vi "Inversion Neighborhood.vi"(8 "w":i32, 9 "y":i32, 10 "Generate Random Indices?":bool, 11 "Schedule in":u16[](array[numeric])) -> (3 "Schedule out":u16[](array[numeric]))   [LabVIEW 2013]
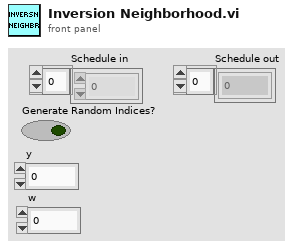
[diagram p1: front panel]
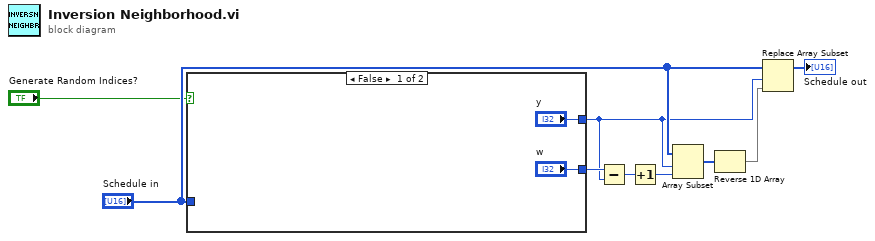
[diagram p0: block diagram]
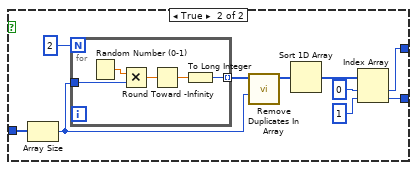
[diagram p2: hidden frame]
diagram:
  n1 = case shown="False" "Generate Random Indices?" {
    tunnel: "Schedule in" -> [_ w21]
    tunnel: ["w" w13] -> w7
    tunnel: ["y" w12] -> w6
    frame False {
    }
    frame True {
      n2 = Array Size(array=w21) -> (size(s)=w18:i32)
      n3 = for {
        N: 2 -> [_]
        tunnel: w18 -> [w23]
        tunnel: [w22] -> w19 mode=indexing
        n4 = Random Number (0-1)() -> (number: 0 to 1=w26:dbl)
        n5 = Multiply(x=w26, y=w23) -> (x*y=w25:dbl)
        n6 = Round Toward -Infinity(1:w25) -> (0:w24:dbl)
        n7 = To Long Integer(number=w24) -> (32bit integer=w22:i32)
      }
      n8 = call "Remove Duplicates In Array.vi"("Max Index Bound"=w18, "Random Numbers Array"=w19) -> ("Random Numbers Array without Duplicates"=w15:i32[])  [unwired: 9 in]
      n9 = Sort 1D Array(array=w15) -> (sorted array=w14:i32[])
      n10 = Index Array(array=w14, index #1=0 ("index"), index #2=1 ("index")) -> (element #1=w12:i32, element #2=w13:i32)
    }
  }
  n11 = Subtract(x=w7, y=w6) -> (x-y=w3:i32)
  n12 = Increment(x=w3) -> (x+1=w2:i32)
  n13 = Array Subset(array="Schedule in", index=w6, length=w2) -> (w5:u16[])
  n14 = Reverse 1D Array(array=w5) -> (reversed array=w4:u16[])
  n15 = Replace Array Subset(array="Schedule in", new element=w4, index=w6) -> (→"Schedule out":u16[])
